vi "ReadBPMProfile.vi"(8 "Error In":errorcluster, 11 "BPM Task In":refnum<k21>) -> (0 "Error Out":errorcluster, 2 "BPM Profile Data":dbl[][](array[numeric]), 3 "BPM Task Out":refnum<k21>)   [LabVIEW 2012]
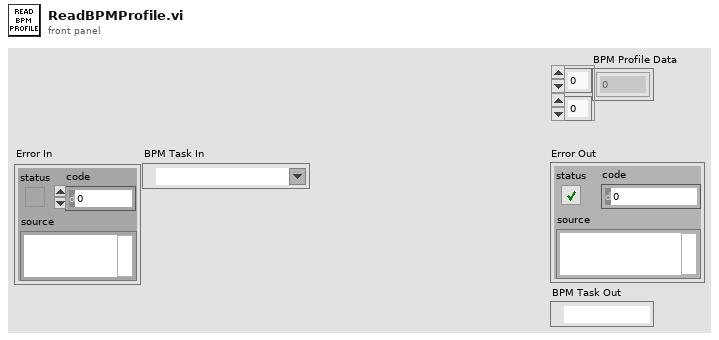
[diagram p1: front panel]
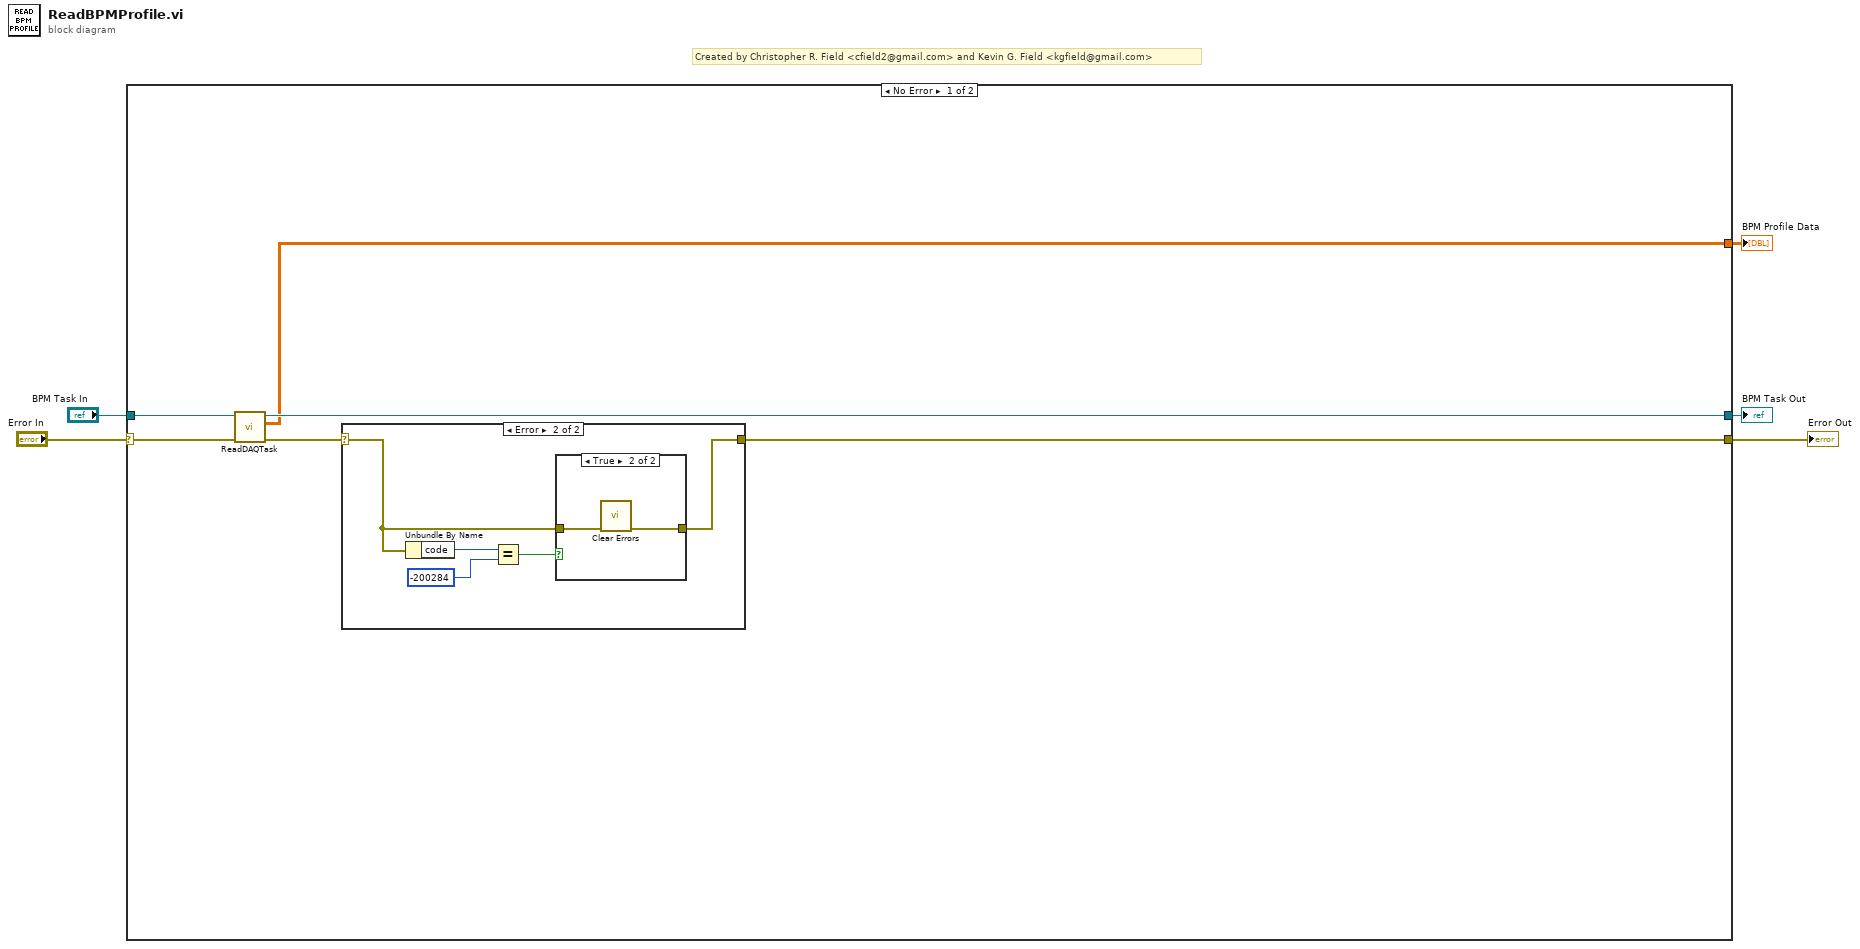
[diagram p0: block diagram]
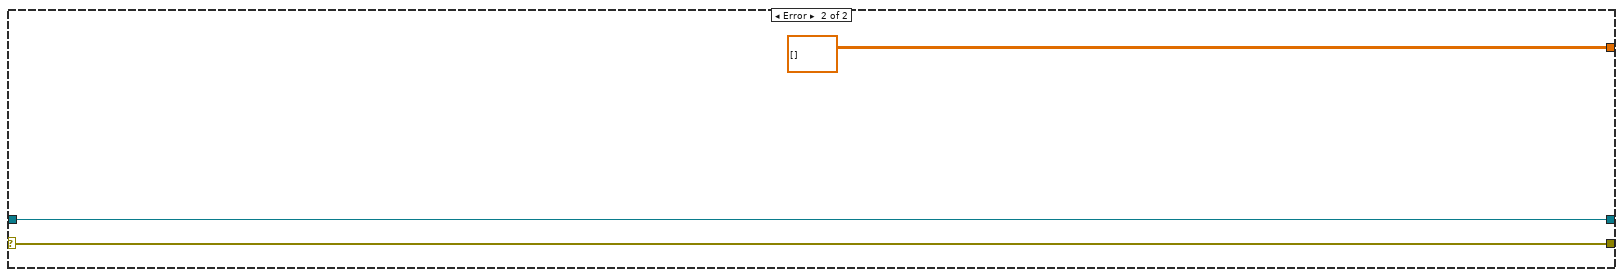
[diagram p4: hidden frame]
diagram:
  # "Created by Christopher R. Field <cfield2@gmail.com> and Kevin G. Field <kgfield@gmail.com>"
  n1 = case shown="No Error" "Error In" {
    selector: "Error In" -> [w8 w22]
    tunnel: "BPM Task In" -> [w9 w23]
    tunnel: [w11 w23] -> w2
    tunnel: [w6 w22] -> w3
    tunnel: [w10 dbl[][] [] ("data")] -> w1
    frame No Error {
      n2 = call "ReadDAQTask.vi"("Error In"=w8, "DAQ Task In"=w9) -> ("Error Out"=w7:errorcluster, "Data"=w10:dbl[][], "DAQ Task Out"=w11:refnum<k21>)  [unwired: 7 in]
      n3 = case shown="Error" w7 {
        selector: w7 -> [w12 w14]
        tunnel: [w12 w13] -> w6
        frame No Error {
        }
        frame Error {
          n4 = Unbundle By Name(w14) -> ("code"=w17:i32)
          n5 = Equal?(x=w17, y=-200284) -> (x = y?=w15:bool)
          n6 = case shown="True" w15 {
            tunnel: w14 -> [w18 w20]
            tunnel: [w18 w19] -> w13
            frame False {
            }
            frame True {
              n7 = call <vilib>:"Clear Errors.vi"("error in (no error)"=w20) -> ("error out"=w19:errorcluster)  [unwired: 6 in]
            }
          }
        }
      }
    }
    frame Error {
    }
  }
  "Error Out" <- w3
  "BPM Task Out" <- w2
  "BPM Profile Data" <- w1
